vi "PriorityQueue Usage Example2.vi"() -> ()   [LabVIEW 2019]
doc: "This is an example illustrates how a priority queue could be used in an application."
uses:
  PriorityQueue/PriorityQueue.lvclass
panel:
  in  "stop":bool
  in  "Wait3":bool
  in  "Wait2":bool
  in  "Wait1":bool
  out "Waits in Queue":dbl[](array[numeric])
  # "This example shows the queue behavior when elements with different priorities are placed on the queue.  The buttons queue up processes that take different amounts of time.  The 0.5 second process is priority 0, the 1.5 second process is priority 1, and the 3 second process is priority 2.\n\nStart the vi and use the buttons to add elements to the queue.  Regardless of the order in which the elements are added to the queue, they are always in priority order on the queue.\n\n(Note:  Only messages currently on the queue are shown.  Since the first message is dequeued immediately, it will not show up in the array indicator.)"
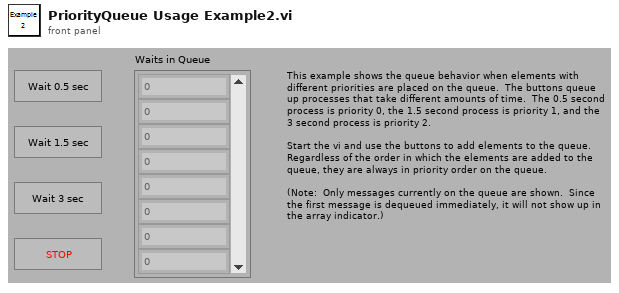
[diagram p1: front panel]
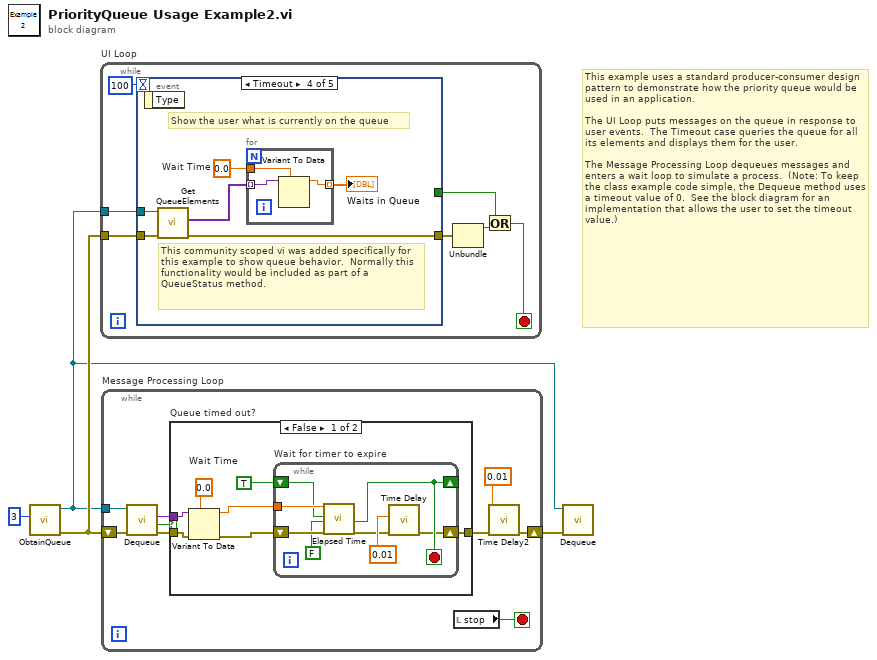
[diagram p0: block diagram]
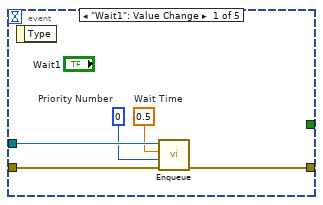
[diagram p3: hidden frame]
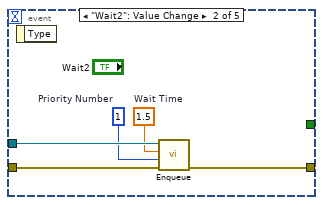
[diagram p4: hidden frame]
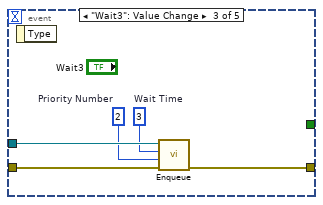
[diagram p5: hidden frame]
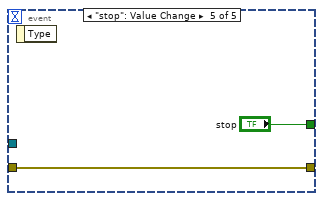
[diagram p6: hidden frame]
diagram:
  # "This example uses a standard producer-consumer design pattern to demonstrate how the priority queue would be used in an application.\n\nThe UI Loop puts messages on the queue in response to user events.  The Timeout case queries the queue for all its elements and displays them for the user.\n\nThe Message Processing Loop dequeues messages and enters a wait loop to simulate a process.  (Note: To keep the class example code simple, the Dequeue method uses a timeout value of 0.  See the block diagram for an implementation that allows the user to set the timeout value.)"
  n1 = call "ObtainQueue.vi"("# Priority Levels (5)"=3) -> ("error out"=w3:errorcluster, "PriorityQueue out"=w1:refnum<class "PriorityQueue.lvclass">)  [unwired: 9 in]
  n2 = while "UI Loop" {
    tunnel: w1 -> [w10]
    tunnel: w3 -> [w11]
    stop <- w6 stop-if-true
    n3 = event shown="[3] Timeout" {
      selector: _ -> [_ _ _ _ _]
      dyn-events: _ -> [_ _ _ _ _]
      timeout: 100 -> [_ _ _ _ _]
      tunnel: w11 -> [w16 w21 w26 w32 w37]
      tunnel: w10 -> [w15 w20 w25 w30 _]
      tunnel: [w12 w17 w22 w31 w37] -> w8
      tunnel: [_ _ _ _ "stop"] -> w5
      event "Wait1": Value Change {
        w13 = 0  # Priority Number
        w14 = 0.5  # Wait Time
        n4 = event-data() -> ()  [unwired: 1 in, 1 out]
        n5 = call-dynamic "Enqueue.vi"("error in (no error)"=w16, "Priority Number"=w13, "Element"=w14, "PriorityQueue in"=w15) -> ("error out"=w12:errorcluster)  [unwired: 6 in, 1 out]
      }
      event "Wait2": Value Change {
        w18 = 1  # Priority Number
        w19 = 1.5  # Wait Time
        n6 = event-data() -> ()  [unwired: 1 in, 1 out]
        n7 = call-dynamic "Enqueue.vi"("error in (no error)"=w21, "Priority Number"=w18, "Element"=w19, "PriorityQueue in"=w20) -> ("error out"=w17:errorcluster)  [unwired: 6 in, 1 out]
      }
      event "Wait3": Value Change {
        w23 = 2  # Priority Number
        w24 = 3  # Wait Time
        n8 = event-data() -> ()  [unwired: 1 in, 1 out]
        n9 = call-dynamic "Enqueue.vi"("error in (no error)"=w26, "Priority Number"=w23, "Element"=w24, "PriorityQueue in"=w25) -> ("error out"=w22:errorcluster)  [unwired: 6 in, 1 out]
      }
      event Timeout {
        w27 = 0.0  # Wait Time
        # "Show the user what is currently on the queue"
        # "This community scoped vi was added specifically for this example to show queue behavior.  Normally this functionality would be included as part of a QueueStatus method."
        n10 = event-data() -> ()  [unwired: 1 in, 1 out]
        n11 = call "Get QueueElements.vi"("error in (no error)"=w32, "PriorityQueue in"=w30) -> ("error out"=w31:errorcluster, "Queue Elements"=w29:variant[])  [unwired: 7 in, 1 out]
        n12 = for {
          tunnel: w29 -> [w35] mode=indexing
          tunnel: [w34] -> w28 mode=indexing
          tunnel: w27 -> [w33]
          n13 = Variant To Data(type=w33, Variant=w35) -> (data=w34:dbl)  [unwired: 1 in, 1 out]
        }
        "Waits in Queue" <- w28
      }
      event "stop": Value Change {
        n14 = event-data() -> ()  [unwired: 1 in, 1 out]
      }
    }
    n15 = Unbundle(w8) -> ("status"=w7:bool)  [unwired: 2 out]
    n16 = Or(x=w5, y=w7) -> (x .or. y?=w6:bool)
  }
  n17 = while "Message Processing Loop" {
    shift-right: [w40] -> w2
    shift-left: w3 -> [w45]
    tunnel: w1 -> [w46]
    stop <- w41 stop-if-true
    n18 = call-dynamic "Dequeue.vi"("error in (no error)"=w45, "PriorityQueue in"=w46) -> ("error out"=w43:errorcluster, "Timed Out?"=w44:bool, "Element"=w42:variant)  [unwired: 6 in, 1 out]
    n19 = case "Queue timed out?" shown="False" w44 {
      tunnel: w43 -> [w52 w62]
      tunnel: w42 -> [w53 _]
      tunnel: [w49 w62] -> w39
      frame False {
        w51 = 0.0  # Wait Time
        n20 = Variant To Data(error in=w52, type=w51, Variant=w53) -> (data=w48:dbl, error out=w50:errorcluster)
        n21 = while "Wait for timer to expire" {
          tunnel: w48 -> [w60]
          shift-right: [w57] -> _
          shift-left: TRUE ("Auto Reset") -> [w58]
          shift-right: [w54] -> w49
          shift-left: w50 -> [w61]
          stop <- w57 stop-if-true
          n22 = call "Elapsed Time"("Time Target (s)"=w60, "Reset"=w58, "Auto Reset"=FALSE, "error in (no error)"=w61) -> ("Time has Elapsed"=w57:bool, "error out"=w55:errorcluster)  [unwired: 8 in, 6 out]
          n23 = call "Time Delay"("error in (no error)"=w55, "Delay Time (s)"=0.01) -> ("error out"=w54:errorcluster)  [unwired: 9 in]
        }
      }
      frame True {
        # "No messages"
      }
    }
    n24 = local read "stop"() -> (w41:bool)
    n25 = call "Time Delay2"("error in (no error)"=w39, "Delay Time (s)"=0.01) -> ("error out"=w40:errorcluster)  [unwired: 9 in]
  }
  n26 = call-dynamic "Dequeue.vi"("error in (no error)"=w2, "PriorityQueue in"=w1) -> ()  [unwired: 6 in, 4 out]
